vi "Close Demosaicker.vi"(8 "error in (no error)":errorcluster, 11 "Demosaicker reference":refnum<k24>) -> (0 "error out":errorcluster)   [LabVIEW 2022 SP3]
uses:
  I:/.shortcut-targets-by-id/1riZacJd_1_jmKfGgrjDuP7KcecvMS3i2/Xiao research group/Programs/XYZRecorrection/Scientific Camera Interfaces/SDK/DotNet Toolkit/dlls/Managed_64_lib/Thorlabs.TSI.Demosaicker.dll
  SDK/DotNet Toolkit/dlls/Managed_64_lib/Thorlabs.TSI.Demosaicker.dll
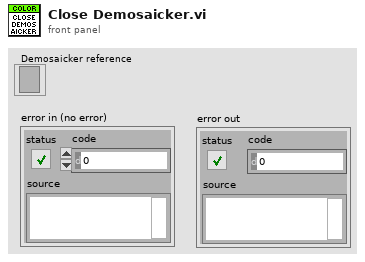
[diagram p1: front panel]
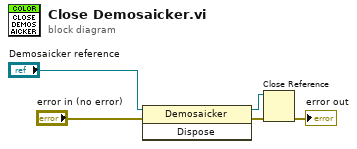
[diagram p0: block diagram]
diagram:
  n1 = invoke class="Demosaicker" method="Dispose"(reference="Demosaicker reference", error in="error in (no error)") -> (reference out=w3:refnum<k24>, error out=w4:errorcluster)  [unwired: 1 in, 1 out]
  n2 = Close Reference(reference=w3, error in (no error)=w4) -> (error out=→"error out":errorcluster)
